vi "Apply.vi"(8 "error in":errorcluster, 11 "DO DAQmx Fixed Freq PWM CFG in":refnum<class "DO DAQmx Fixed Freq PWM CFG.lvclass">) -> (0 "error out":errorcluster, 3 "DO DAQmx Fixed Freq PWM CFG out":refnum<class "DO DAQmx Fixed Freq PWM CFG.lvclass">)   [LabVIEW 2024, in "DO DAQmx Fixed Freq PWM CFG.lvclass"]
uses:
  DO DAQmx Fixed Freq PWM CFG.lvclass
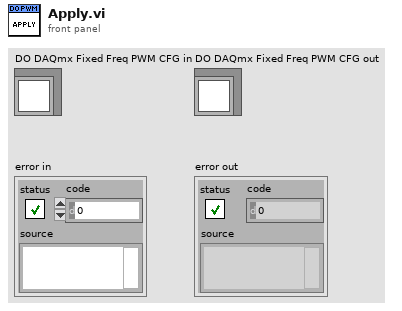
[diagram p1: front panel]
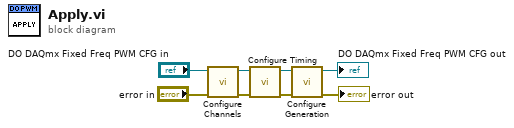
[diagram p0: block diagram]
diagram:
  n1 = call-dynamic "Configure Channels.vi"("error in"="error in", "DO DAQmx Fixed Freq PWM CFG in"="DO DAQmx Fixed Freq PWM CFG in") -> ("error out"=w7:errorcluster, "DO DAQmx Fixed Freq PWM CFG out"=w8:refnum<class "DO DAQmx Fixed Freq PWM CFG.lvclass">)  [unwired: 8 in]
  n2 = call-dynamic "Configure Timing.vi"("error in"=w7, "DAQmx Base CFG in"=w8) -> ("error out"=w5:errorcluster, "DAQmx Base CFG out"=w2:refnum<class "DO DAQmx Fixed Freq PWM CFG.lvclass">)  [unwired: 8 in]
  n3 = call-dynamic "Configure Generation.vi"("error in"=w5, "DO DAQmx Fixed Freq PWM CFG in"=w2) -> ("error out"=→"error out":errorcluster, "DO DAQmx Fixed Freq PWM CFG out"=→"DO DAQmx Fixed Freq PWM CFG out":refnum<class "DO DAQmx Fixed Freq PWM CFG.lvclass">)  [unwired: 8 in]
